vi "输入数据解析.vi"(0 "单个参数补充":dbl, 1 "从板号":dbl=1.0, 2 "主板二维码":string="BNET01", 3 "从板二维码":string="BNET01", 5 "主板引用":refnum<vi>, 7 "从板引用":refnum<vi>, 9 "主板选项":string="三级故障阀值", 11 "枚举":enum16{"主板", "从板"}(ring), 12 "快换":bool caption="快换写入") -> (4 "输出数组":dbl[][](array[numeric]), 6 "数组长度":dbl[](array[numeric]), 8 "循环次数":i32, 10 "命令":u32, 14 "名称":string[](array[string]), 15 "命令序号":u32[](array[numeric]))   [LabVIEW 2013] (continued)
                  frame "8", "钛酸锂" {
                  }
                  frame "9", "其他电池" {
                  }
                  frame "1", "磷酸铁锂", Default {
                  }
                }
                n5418 = Match Pattern(string=w14174, regular expression=w14173) -> (before substring=w14172:string, after substring=w14171:string)  [unwired: 3 out]
                n5419 = call "输入分辨率计算-EV05.vi"("1字节?"=FALSE, "数值"=w14211, "分辨率"=0.1) -> ("低字节"=w14182:dbl, "高字节1"=w14183:dbl)  [unwired: 2 in, 5 out]
                n5420 = Quotient & Remainder(x=w14190, y=w14205) -> (x-y*floor(x/y)=w14204:dbl, floor(x/y)=w14208:dbl)
                n5421 = Fract/Exp String To Number(string=w14175) -> (number=w14166:dbl)  [unwired: 4 out]
                n5422 = Quotient & Remainder(x=w14189, y=w14200) -> (x-y*floor(x/y)=w14196:dbl, floor(x/y)=w14197:dbl)
                n5423 = Quotient & Remainder(x=w14208, y=w14205) -> (x-y*floor(x/y)=w14203:dbl, floor(x/y)=w14207:dbl)
                n5424 = Fract/Exp String To Number(string=w14172) -> (number=w14165:dbl)  [unwired: 4 out]
                n5425 = Quotient & Remainder(x=w14197, y=w14200) -> (x-y*floor(x/y)=w14195:dbl, floor(x/y)=w14198:dbl)
                n5426 = call <vilib>:"Trim Whitespace.vi"("string"=w14171) -> ("trimmed string"=w14170:string)  [unwired: 1 in]
                n5427 = Quotient & Remainder(x=w14207, y=w14205) -> (x-y*floor(x/y)=w14202:dbl, floor(x/y)=w14206:dbl)
                n5428 = Quotient & Remainder(x=w14198, y=w14200) -> (x-y*floor(x/y)=w14194:dbl, floor(x/y)=w14199:dbl)
                n5429 = Quotient & Remainder(x=w14229, y=256.0) -> (x-y*floor(x/y)=w14231:dbl, floor(x/y)=w14232:dbl)
                n5430 = Fract/Exp String To Number(string=w14170) -> (number=w14164:dbl)  [unwired: 4 out]
                n5431 = Quotient & Remainder(x=w14206, y=w14205) -> (x-y*floor(x/y)=w14201:dbl)  [unwired: 1 out]
                n5432 = Quotient & Remainder(x=w14199, y=w14200) -> (x-y*floor(x/y)=w14193:dbl)  [unwired: 1 out]
                n5433 = Build Array(w14184, w14185, w14201, w14202, w14203, w14204, w14193, w14194, w14195, w14196, w14183, w14182, w14181, w14181, w14181, w14169, w14168, w14167, w14166, w14165, w14164) -> (w14180:dbl[])
                n5434 = Build Array(w14232, w14231, w14228, w14226, w14224) -> (w14230:dbl[])
                n5435 = Insert Into Array(array=w14230, new element=w14180) -> (w14213:dbl[])  [unwired: 1 in]
              }
              frame 1 {
                w14258 = 256.0 ("y")
                n5436 = Unbundle By Name(w14248) -> ("电池包组号"=w14259:string)
                n5437 = Decimal String To Number(string=w14259, default (0L)=0.0) -> (number=w14254:dbl)  [unwired: 1 in, 1 out]
                n5438 = Quotient & Remainder(x=w14254, y=w14258) -> (x-y*floor(x/y)=w14249:dbl, floor(x/y)=w14255:dbl)
                n5439 = Quotient & Remainder(x=w14255, y=w14258) -> (x-y*floor(x/y)=w14250:dbl, floor(x/y)=w14256:dbl)
                n5440 = Quotient & Remainder(x=w14256, y=w14258) -> (x-y*floor(x/y)=w14251:dbl, floor(x/y)=w14257:dbl)
                n5441 = Quotient & Remainder(x=w14257, y=w14258) -> (x-y*floor(x/y)=w14252:dbl)  [unwired: 1 out]
                n5442 = Build Array(w14252, w14251, w14250, w14249) -> (w14247:dbl[])
              }
              frame 2 {
                w14278 = 256.0 ("y")
                w14283 = 256.0 ("y")
                n5443 = Unbundle By Name(w14270) -> ("累计充电总安时"=w14267:dbl, "累计放电总安时"=w14266:dbl)
                n5444 = call "输入分辨率计算-EV05.vi"("1字节?"=TRUE, "数值 2"=w14266, "数值"=w14267, "分辨率"=0.001) -> ("高字节 2"=w14264:dbl, "高字节1"=w14265:dbl)  [unwired: 1 in, 5 out]
                n5445 = Quotient & Remainder(x=w14265, y=w14283) -> (x-y*floor(x/y)=w14282:dbl, floor(x/y)=w14286:dbl)
                n5446 = Quotient & Remainder(x=w14264, y=w14278) -> (x-y*floor(x/y)=w14274:dbl, floor(x/y)=w14275:dbl)
                n5447 = Quotient & Remainder(x=w14286, y=w14283) -> (x-y*floor(x/y)=w14281:dbl, floor(x/y)=w14285:dbl)
                n5448 = Quotient & Remainder(x=w14275, y=w14278) -> (x-y*floor(x/y)=w14273:dbl, floor(x/y)=w14276:dbl)
                n5449 = Quotient & Remainder(x=w14285, y=w14283) -> (x-y*floor(x/y)=w14280:dbl, floor(x/y)=w14284:dbl)
                n5450 = Quotient & Remainder(x=w14276, y=w14278) -> (x-y*floor(x/y)=w14272:dbl, floor(x/y)=w14277:dbl)
                n5451 = Quotient & Remainder(x=w14284, y=w14283) -> (x-y*floor(x/y)=w14279:dbl)  [unwired: 1 out]
                n5452 = Quotient & Remainder(x=w14277, y=w14278) -> (x-y*floor(x/y)=w14271:dbl)  [unwired: 1 out]
                n5453 = Build Array(w14279, w14280, w14281, w14282, w14271, w14272, w14273, w14274) -> (w14287:dbl[])
              }
              frame 3 {
                w14299 = 256.0 ("y")
                n5454 = Unbundle By Name(w14294) -> ("电池放空次数"=w14293:dbl, "电池充满次数"=w14292:dbl, "电池充电次数"=w14291:dbl)
                n5455 = Quotient & Remainder(x=w14293, y=w14299) -> (x-y*floor(x/y)=w14301:dbl, floor(x/y)=w14302:dbl)
                n5456 = Quotient & Remainder(x=w14292, y=w14299) -> (x-y*floor(x/y)=w14297:dbl, floor(x/y)=w14298:dbl)
                n5457 = Quotient & Remainder(x=w14291, y=w14299) -> (x-y*floor(x/y)=w14295:dbl, floor(x/y)=w14296:dbl)
                n5458 = Build Array(w14302, w14301, w14298, w14297, w14296, w14295) -> (w14300:dbl[])
              }
            }
          }
        }
        frame "电池包组号" {
          n5459 = Unbundle By Name(w14308) -> ("电池信息"=w14309:refnum<vi>)
          n5460 = property class="Clust (严格)"(reference=w14309) -> ("Value"=w14307:T7)  [unwired: 1 in, 2 out]
          n5461 = for {
            N: 1 -> [_]
            tunnel: [w14319] -> w14313 mode=indexing
            tunnel: [w14318] -> w14312 mode=indexing
            tunnel: [w14316] -> w14310 mode=indexing
            tunnel: w14307 -> [w14315]
            i -> [w14317]
            n5462 = case shown="0, 默认" w14317 {
              tunnel: [4 ("单个参数补充") 30 ("单个参数补充") 8 ("单个参数补充") 6 ("单个参数补充")] -> w14319
              tunnel: [2 ("命令序号") 1 ("命令序号") 4 ("命令序号") 5 ("命令序号")] -> w14318
              tunnel: [w14332 w14337 w14425 w14437] -> w14316
              tunnel: w14315 -> [w14331 w14346 w14408 w14431]
              frame 0, Default {
                w14329 = 256.0 ("y")
                n5463 = Unbundle By Name(w14331) -> ("电池包组号"=w14330:string)
                n5464 = Decimal String To Number(string=w14330, default (0L)=0.0) -> (number=w14325:dbl)  [unwired: 1 in, 1 out]
                n5465 = Quotient & Remainder(x=w14325, y=w14329) -> (x-y*floor(x/y)=w14320:dbl, floor(x/y)=w14326:dbl)
                n5466 = Quotient & Remainder(x=w14326, y=w14329) -> (x-y*floor(x/y)=w14321:dbl, floor(x/y)=w14327:dbl)
                n5467 = Quotient & Remainder(x=w14327, y=w14329) -> (x-y*floor(x/y)=w14322:dbl, floor(x/y)=w14328:dbl)
                n5468 = Quotient & Remainder(x=w14328, y=w14329) -> (x-y*floor(x/y)=w14323:dbl)  [unwired: 1 out]
                n5469 = Build Array(w14323, w14322, w14321, w14320) -> (w14332:dbl[])
              }
              frame 1 {
                w14359 = 2 ("偏移量(0)")
                w14356 = "-" ("正则表达式")
                n5470 = Unbundle By Name(w14346) -> ("电池包额定容量"=w14353:dbl, "电池包额定能量"=w14352:dbl, "电池包额定总电压"=w14347:dbl, "实际容量"=w14335:dbl)
                n5471 = Unbundle By Name(w14346) -> ("电池串联"=w14367:dbl, "电池并联"=w14366:dbl, "电池厂家"=w14365:string, "电池类型"=w14363:string, "电池生产日期"=w14361:string)
                n5472 = Match Pattern(string=w14361, regular expression=w14356) -> (before substring=w14360:string, after substring=w14357:string)  [unwired: 3 out]
                n5473 = Match Pattern(string=w14357, regular expression=w14356) -> (before substring=w14355:string, after substring=w14354:string)  [unwired: 3 out]
                n5474 = String Subset(string=w14360, offset (0)=w14359, length (rest)=w14359) -> (substring=w14358:string)
                n5475 = case shown="\"2\", \"盟固利\"" w14365 {
                  tunnel: [2 1] -> w14364
                  frame "2", "盟固利" {
                  }
                  frame "1", "普莱德", Default {
                  }
                }
                n5476 = case shown="\"9\", \"其他电池\"" w14363 {
                  tunnel: [2 3 4 5 6 7 8 9 1] -> w14362
                  frame "2", "锰酸锂" {
                  }
                  frame "3", "三元材料" {
                  }
                  frame "4", "铅酸" {
                  }
                  frame "5", "镍氢" {
                  }
                  frame "6", "钴酸锂" {
                  }
                  frame "7", "聚合物锂离子" {
                  }
                  frame "8", "钛酸锂" {
                  }
                  frame "9", "其他电池" {
                  }
                  frame "1", "磷酸铁锂", Default {
                  }
                }
                n5477 = call "输入分辨率计算-EV05.vi"("1字节?"=FALSE, "数值 2"=w14352, "数值"=w14353, "分辨率"=0.1) -> ("低字节 2"=w14342:dbl, "高字节 2"=w14343:dbl, "低字节"=w14344:dbl, "高字节1"=w14345:dbl)  [unwired: 1 in, 3 out]
                n5478 = call "输入分辨率计算-EV05.vi"("1字节?"=FALSE, "数值 2"=w14335, "数值"=w14347, "分辨率"=0.1) -> ("低字节 2"=w14338:dbl, "高字节 2"=w14339:dbl, "低字节"=w14340:dbl, "高字节1"=w14341:dbl)  [unwired: 1 in, 3 out]
                n5479 = Fract/Exp String To Number(string=w14358) -> (number=w14384:dbl)  [unwired: 1 in, 3 out]
                n5480 = Fract/Exp String To Number(string=w14355) -> (number=w14382:dbl)  [unwired: 4 out]
                n5481 = Fract/Exp String To Number(string=w14354) -> (number=w14380:dbl)  [unwired: 4 out]
                n5482 = Build Array(w14345, w14344, w14343, w14342, w14341, w14340, w14339, w14338) -> (w14336:dbl[])
                n5483 = Quotient & Remainder(x=w14367, y=256.0) -> (x-y*floor(x/y)=w14386:dbl, floor(x/y)=w14387:dbl)
                n5484 = call "二进制解析-8.6.vi"("索引"=7, "数值"=w14384) -> ("低位子数组"=w14375:i32[])  [unwired: 3 out]
                n5485 = call "二进制解析-8.6.vi"("索引"=4, "数值"=w14382) -> ("低位子数组"=w14378:i32[])  [unwired: 3 out]
                n5486 = call "二进制解析-8.6.vi"("索引"=5, "数值"=w14380) -> ("低位子数组"=w14372:i32[])  [unwired: 3 out]
                n5487 = Delete From Array(array=w14378, length=1 ("长度"), index=0 ("索引")) -> (deleted portion=w14374:i32[], array with subset deleted=w14373:i32[])
                n5488 = Insert Into Array(array=w14375, new element=w14374) -> (w14371:i32[])  [unwired: 1 in]
                n5489 = Insert Into Array(array=w14373, new element=w14372) -> (w14370:i32[])  [unwired: 1 in]
                n5490 = call "数值二进制转十进制-8.6.vi"("子数组"=w14371) -> ("十进制数值"=w14369:i32)  [unwired: 4 out]
                n5491 = call "数值二进制转十进制-8.6.vi"("子数组"=w14370) -> ("十进制数值"=w14368:i32)  [unwired: 4 out]
                n5492 = Build Array(w14387, w14386, w14366, w14364, w14362, w14369, w14368) -> (w14385:dbl[])
                n5493 = Insert Into Array(array=w14385, new element=w14336) -> (w14337:dbl[])  [unwired: 1 in]
              }
              frame 3 {
                w14416 = 256.0 ("y")
                w14421 = 256.0 ("y")
                n5494 = Unbundle By Name(w14408) -> ("累计充电总安时"=w14405:dbl, "累计放电总安时"=w14404:dbl)
                n5495 = call "输入分辨率计算-EV05.vi"("1字节?"=TRUE, "数值 2"=w14404, "数值"=w14405, "分辨率"=0.001) -> ("高字节 2"=w14402:dbl, "高字节1"=w14403:dbl)  [unwired: 1 in, 5 out]
                n5496 = Quotient & Remainder(x=w14403, y=w14421) -> (x-y*floor(x/y)=w14420:dbl, floor(x/y)=w14424:dbl)
                n5497 = Quotient & Remainder(x=w14402, y=w14416) -> (x-y*floor(x/y)=w14412:dbl, floor(x/y)=w14413:dbl)
                n5498 = Quotient & Remainder(x=w14424, y=w14421) -> (x-y*floor(x/y)=w14419:dbl, floor(x/y)=w14423:dbl)
                n5499 = Quotient & Remainder(x=w14413, y=w14416) -> (x-y*floor(x/y)=w14411:dbl, floor(x/y)=w14414:dbl)
                n5500 = Quotient & Remainder(x=w14423, y=w14421) -> (x-y*floor(x/y)=w14418:dbl, floor(x/y)=w14422:dbl)
                n5501 = Quotient & Remainder(x=w14414, y=w14416) -> (x-y*floor(x/y)=w14410:dbl, floor(x/y)=w14415:dbl)
                n5502 = Quotient & Remainder(x=w14422, y=w14421) -> (x-y*floor(x/y)=w14417:dbl)  [unwired: 1 out]
                n5503 = Quotient & Remainder(x=w14415, y=w14416) -> (x-y*floor(x/y)=w14409:dbl)  [unwired: 1 out]
                n5504 = Build Array(w14417, w14418, w14419, w14420, w14409, w14410, w14411, w14412) -> (w14425:dbl[])
              }
              frame 4 {
                w14436 = 256.0 ("y")
                n5505 = Unbundle By Name(w14431) -> ("电池放空次数"=w14430:dbl, "电池充满次数"=w14429:dbl, "电池充电次数"=w14428:dbl)
                n5506 = Quotient & Remainder(x=w14430, y=w14436) -> (x-y*floor(x/y)=w14438:dbl, floor(x/y)=w14439:dbl)
                n5507 = Quotient & Remainder(x=w14429, y=w14436) -> (x-y*floor(x/y)=w14434:dbl, floor(x/y)=w14435:dbl)
                n5508 = Quotient & Remainder(x=w14428, y=w14436) -> (x-y*floor(x/y)=w14432:dbl, floor(x/y)=w14433:dbl)
                n5509 = Build Array(w14439, w14438, w14435, w14434, w14433, w14432) -> (w14437:dbl[])
              }
            }
          }
        }
        frame "充放电安时" {
          n5510 = Unbundle By Name(w14445) -> ("电池信息"=w14446:refnum<vi>)
          n5511 = property class="Clust (严格)"(reference=w14446) -> ("Value"=w14444:T7)  [unwired: 1 in, 2 out]
          n5512 = for {
            N: 1 -> [_]
            tunnel: [w14456] -> w14450 mode=indexing
            tunnel: [w14455] -> w14449 mode=indexing
            tunnel: [w14453] -> w14447 mode=indexing
            tunnel: w14444 -> [w14452]
            i -> [w14454]
            n5513 = case shown="0, 默认" w14454 {
              tunnel: [8 ("单个参数补充") 30 ("单个参数补充") 4 ("单个参数补充") 6 ("单个参数补充")] -> w14456
              tunnel: [3 ("命令序号") 1 ("命令序号") 2 ("命令序号") 5 ("命令序号")] -> w14455
              tunnel: [w14480 w14485 w14562 w14574] -> w14453
              tunnel: w14452 -> [w14463 w14494 w14561 w14568]
              frame 0, Default {
                w14471 = 256.0 ("y")
                w14476 = 256.0 ("y")
                n5514 = Unbundle By Name(w14463) -> ("累计充电总安时"=w14460:dbl, "累计放电总安时"=w14459:dbl)
                n5515 = call "输入分辨率计算-EV05.vi"("1字节?"=TRUE, "数值 2"=w14459, "数值"=w14460, "分辨率"=0.001) -> ("高字节 2"=w14457:dbl, "高字节1"=w14458:dbl)  [unwired: 1 in, 5 out]
                n5516 = Quotient & Remainder(x=w14458, y=w14476) -> (x-y*floor(x/y)=w14475:dbl, floor(x/y)=w14479:dbl)
                n5517 = Quotient & Remainder(x=w14457, y=w14471) -> (x-y*floor(x/y)=w14467:dbl, floor(x/y)=w14468:dbl)
                n5518 = Quotient & Remainder(x=w14479, y=w14476) -> (x-y*floor(x/y)=w14474:dbl, floor(x/y)=w14478:dbl)
                n5519 = Quotient & Remainder(x=w14468, y=w14471) -> (x-y*floor(x/y)=w14466:dbl, floor(x/y)=w14469:dbl)
                n5520 = Quotient & Remainder(x=w14478, y=w14476) -> (x-y*floor(x/y)=w14473:dbl, floor(x/y)=w14477:dbl)
                n5521 = Quotient & Remainder(x=w14469, y=w14471) -> (x-y*floor(x/y)=w14465:dbl, floor(x/y)=w14470:dbl)
                n5522 = Quotient & Remainder(x=w14477, y=w14476) -> (x-y*floor(x/y)=w14472:dbl)  [unwired: 1 out]
                n5523 = Quotient & Remainder(x=w14470, y=w14471) -> (x-y*floor(x/y)=w14464:dbl)  [unwired: 1 out]
                n5524 = Build Array(w14472, w14473, w14474, w14475, w14464, w14465, w14466, w14467) -> (w14480:dbl[])
              }
              frame 1 {
                w14507 = 2 ("偏移量(0)")
                w14504 = "-" ("正则表达式")
                n5525 = Unbundle By Name(w14494) -> ("电池包额定容量"=w14501:dbl, "电池包额定能量"=w14500:dbl, "电池包额定总电压"=w14495:dbl, "实际容量"=w14483:dbl)
                n5526 = Unbundle By Name(w14494) -> ("电池串联"=w14515:dbl, "电池并联"=w14514:dbl, "电池厂家"=w14513:string, "电池类型"=w14511:string, "电池生产日期"=w14509:string)
                n5527 = Match Pattern(string=w14509, regular expression=w14504) -> (before substring=w14508:string, after substring=w14505:string)  [unwired: 3 out]
                n5528 = Match Pattern(string=w14505, regular expression=w14504) -> (before substring=w14503:string, after substring=w14502:string)  [unwired: 3 out]
                n5529 = String Subset(string=w14508, offset (0)=w14507, length (rest)=w14507) -> (substring=w14506:string)
                n5530 = case shown="\"2\", \"盟固利\"" w14513 {
                  tunnel: [2 1] -> w14512
                  frame "2", "盟固利" {
                  }
                  frame "1", "普莱德", Default {
                  }
                }
                n5531 = case shown="\"9\", \"其他电池\"" w14511 {
                  tunnel: [2 3 4 5 6 7 8 9 1] -> w14510
                  frame "2", "锰酸锂" {
                  }
                  frame "3", "三元材料" {
                  }
                  frame "4", "铅酸" {
                  }
                  frame "5", "镍氢" {
                  }
                  frame "6", "钴酸锂" {
                  }
                  frame "7", "聚合物锂离子" {
                  }
                  frame "8", "钛酸锂" {
                  }
                  frame "9", "其他电池" {
                  }
                  frame "1", "磷酸铁锂", Default {
                  }
                }
                n5532 = call "输入分辨率计算-EV05.vi"("1字节?"=FALSE, "数值 2"=w14500, "数值"=w14501, "分辨率"=0.1) -> ("低字节 2"=w14490:dbl, "高字节 2"=w14491:dbl, "低字节"=w14492:dbl, "高字节1"=w14493:dbl)  [unwired: 1 in, 3 out]
                n5533 = call "输入分辨率计算-EV05.vi"("1字节?"=FALSE, "数值 2"=w14483, "数值"=w14495, "分辨率"=0.1) -> ("低字节 2"=w14486:dbl, "高字节 2"=w14487:dbl, "低字节"=w14488:dbl, "高字节1"=w14489:dbl)  [unwired: 1 in, 3 out]
                n5534 = Fract/Exp String To Number(string=w14506) -> (number=w14532:dbl)  [unwired: 1 in, 3 out]
                n5535 = Fract/Exp String To Number(string=w14503) -> (number=w14530:dbl)  [unwired: 4 out]
                n5536 = Fract/Exp String To Number(string=w14502) -> (number=w14528:dbl)  [unwired: 4 out]
                n5537 = Build Array(w14493, w14492, w14491, w14490, w14489, w14488, w14487, w14486) -> (w14484:dbl[])
                n5538 = Quotient & Remainder(x=w14515, y=256.0) -> (x-y*floor(x/y)=w14534:dbl, floor(x/y)=w14535:dbl)
                n5539 = call "二进制解析-8.6.vi"("索引"=7, "数值"=w14532) -> ("低位子数组"=w14523:i32[])  [unwired: 3 out]
                n5540 = call "二进制解析-8.6.vi"("索引"=4, "数值"=w14530) -> ("低位子数组"=w14526:i32[])  [unwired: 3 out]
                n5541 = call "二进制解析-8.6.vi"("索引"=5, "数值"=w14528) -> ("低位子数组"=w14520:i32[])  [unwired: 3 out]
                n5542 = Delete From Array(array=w14526, length=1 ("长度"), index=0 ("索引")) -> (deleted portion=w14522:i32[], array with subset deleted=w14521:i32[])
                n5543 = Insert Into Array(array=w14523, new element=w14522) -> (w14519:i32[])  [unwired: 1 in]
                n5544 = Insert Into Array(array=w14521, new element=w14520) -> (w14518:i32[])  [unwired: 1 in]
                n5545 = call "数值二进制转十进制-8.6.vi"("子数组"=w14519) -> ("十进制数值"=w14517:i32)  [unwired: 4 out]
                n5546 = call "数值二进制转十进制-8.6.vi"("子数组"=w14518) -> ("十进制数值"=w14516:i32)  [unwired: 4 out]
                n5547 = Build Array(w14535, w14534, w14514, w14512, w14510, w14517, w14516) -> (w14533:dbl[])
                n5548 = Insert Into Array(array=w14533, new element=w14484) -> (w14485:dbl[])  [unwired: 1 in]
              }
              frame 3 {
                w14555 = 256.0 ("y")
                n5549 = Unbundle By Name(w14561) -> ("电池包组号"=w14560:string)
                n5550 = Match Pattern(string=w14560, regular expression="-" ("正则表达式")) -> (before substring=w14558:string, after substring=w14557:string)  [unwired: 3 out]
                n5551 = Fract/Exp String To Number(string=w14558) -> (number=w14556:dbl)  [unwired: 1 in, 3 out]
                n5552 = Fract/Exp String To Number(string=w14557) -> (number=w14554:dbl)  [unwired: 4 out]
                n5553 = Quotient & Remainder(x=w14554, y=w14555) -> (x-y*floor(x/y)=w14552:dbl, floor(x/y)=w14553:dbl)
                n5554 = Quotient & Remainder(x=w14556, y=w14555) -> (x-y*floor(x/y)=w14550:dbl, floor(x/y)=w14551:dbl)
                n5555 = Build Array(w14553, w14552, w14551, w14550) -> (w14562:dbl[])
              }
              frame 4 {
                w14573 = 256.0 ("y")
                n5556 = Unbundle By Name(w14568) -> ("电池放空次数"=w14567:dbl, "电池充满次数"=w14566:dbl, "电池充电次数"=w14565:dbl)
                n5557 = Quotient & Remainder(x=w14567, y=w14573) -> (x-y*floor(x/y)=w14575:dbl, floor(x/y)=w14576:dbl)
                n5558 = Quotient & Remainder(x=w14566, y=w14573) -> (x-y*floor(x/y)=w14571:dbl, floor(x/y)=w14572:dbl)
                n5559 = Quotient & Remainder(x=w14565, y=w14573) -> (x-y*floor(x/y)=w14569:dbl, floor(x/y)=w14570:dbl)
                n5560 = Build Array(w14576, w14575, w14572, w14571, w14570, w14569) -> (w14574:dbl[])
              }
            }
          }
        }
        frame "电池充放电次数" {
          n5561 = Unbundle By Name(w14582) -> ("电池信息"=w14583:refnum<vi>)
          n5562 = property class="Clust (严格)"(reference=w14583) -> ("Value"=w14581:T7)  [unwired: 1 in, 2 out]
          n5563 = for {
            N: 1 -> [_]
            tunnel: [w14593] -> w14587 mode=indexing
            tunnel: [w14592] -> w14586 mode=indexing
            tunnel: [w14590] -> w14584 mode=indexing
            tunnel: w14581 -> [w14589]
            i -> [w14591]
            n5564 = case shown="0, 默认" w14591 {
              tunnel: [6 ("单个参数补充") 30 ("单个参数补充") 4 ("单个参数补充") 8 ("单个参数补充")] -> w14593
              tunnel: [4 ("命令序号") 1 ("命令序号") 2 ("命令序号") 3 ("命令序号")] -> w14592
              tunnel: [w14603 w14610 w14687 w14713] -> w14590
              tunnel: w14589 -> [w14597 w14619 w14686 w14696]
              frame 0, Default {
                w14602 = 256.0 ("y")
                n5565 = Unbundle By Name(w14597) -> ("电池放空次数"=w14596:dbl, "电池充满次数"=w14595:dbl, "电池充电次数"=w14594:dbl)
                n5566 = Quotient & Remainder(x=w14596, y=w14602) -> (x-y*floor(x/y)=w14604:dbl, floor(x/y)=w14605:dbl)
                n5567 = Quotient & Remainder(x=w14595, y=w14602) -> (x-y*floor(x/y)=w14600:dbl, floor(x/y)=w14601:dbl)
                n5568 = Quotient & Remainder(x=w14594, y=w14602) -> (x-y*floor(x/y)=w14598:dbl, floor(x/y)=w14599:dbl)
                n5569 = Build Array(w14605, w14604, w14601, w14600, w14599, w14598) -> (w14603:dbl[])
              }
              frame 1 {
                w14632 = 2 ("偏移量(0)")
                w14629 = "-" ("正则表达式")
                n5570 = Unbundle By Name(w14619) -> ("电池包额定容量"=w14626:dbl, "电池包额定能量"=w14625:dbl, "电池包额定总电压"=w14620:dbl, "实际容量"=w14608:dbl)
                n5571 = Unbundle By Name(w14619) -> ("电池串联"=w14640:dbl, "电池并联"=w14639:dbl, "电池厂家"=w14638:string, "电池类型"=w14636:string, "电池生产日期"=w14634:string)
                n5572 = Match Pattern(string=w14634, regular expression=w14629) -> (before substring=w14633:string, after substring=w14630:string)  [unwired: 3 out]
                n5573 = Match Pattern(string=w14630, regular expression=w14629) -> (before substring=w14628:string, after substring=w14627:string)  [unwired: 3 out]
                n5574 = String Subset(string=w14633, offset (0)=w14632, length (rest)=w14632) -> (substring=w14631:string)
                n5575 = case shown="\"2\", \"盟固利\"" w14638 {
                  tunnel: [2 1] -> w14637
                  frame "2", "盟固利" {
                  }
                  frame "1", "普莱德", Default {
                  }
                }
                n5576 = case shown="\"9\", \"其他电池\"" w14636 {
                  tunnel: [2 3 4 5 6 7 8 9 1] -> w14635
                  frame "2", "锰酸锂" {
                  }
                  frame "3", "三元材料" {
                  }
                  frame "4", "铅酸" {
                  }
                  frame "5", "镍氢" {
                  }
                  frame "6", "钴酸锂" {
                  }
                  frame "7", "聚合物锂离子" {
                  }
                  frame "8", "钛酸锂" {
                  }
                  frame "9", "其他电池" {
                  }
                  frame "1", "磷酸铁锂", Default {
                  }
                }
                n5577 = call "输入分辨率计算-EV05.vi"("1字节?"=FALSE, "数值 2"=w14625, "数值"=w14626, "分辨率"=0.1) -> ("低字节 2"=w14615:dbl, "高字节 2"=w14616:dbl, "低字节"=w14617:dbl, "高字节1"=w14618:dbl)  [unwired: 1 in, 3 out]
                n5578 = call "输入分辨率计算-EV05.vi"("1字节?"=FALSE, "数值 2"=w14608, "数值"=w14620, "分辨率"=0.1) -> ("低字节 2"=w14611:dbl, "高字节 2"=w14612:dbl, "低字节"=w14613:dbl, "高字节1"=w14614:dbl)  [unwired: 1 in, 3 out]
                n5579 = Fract/Exp String To Number(string=w14631) -> (number=w14657:dbl)  [unwired: 1 in, 3 out]
                n5580 = Fract/Exp String To Number(string=w14628) -> (number=w14655:dbl)  [unwired: 4 out]
                n5581 = Fract/Exp String To Number(string=w14627) -> (number=w14653:dbl)  [unwired: 4 out]
                n5582 = Build Array(w14618, w14617, w14616, w14615, w14614, w14613, w14612, w14611) -> (w14609:dbl[])
                n5583 = Quotient & Remainder(x=w14640, y=256.0) -> (x-y*floor(x/y)=w14659:dbl, floor(x/y)=w14660:dbl)
                n5584 = call "二进制解析-8.6.vi"("索引"=7, "数值"=w14657) -> ("低位子数组"=w14648:i32[])  [unwired: 3 out]
                n5585 = call "二进制解析-8.6.vi"("索引"=4, "数值"=w14655) -> ("低位子数组"=w14651:i32[])  [unwired: 3 out]
                n5586 = call "二进制解析-8.6.vi"("索引"=5, "数值"=w14653) -> ("低位子数组"=w14645:i32[])  [unwired: 3 out]
                n5587 = Delete From Array(array=w14651, length=1 ("长度"), index=0 ("索引")) -> (deleted portion=w14647:i32[], array with subset deleted=w14646:i32[])
                n5588 = Insert Into Array(array=w14648, new element=w14647) -> (w14644:i32[])  [unwired: 1 in]
                n5589 = Insert Into Array(array=w14646, new element=w14645) -> (w14643:i32[])  [unwired: 1 in]
                n5590 = call "数值二进制转十进制-8.6.vi"("子数组"=w14644) -> ("十进制数值"=w14642:i32)  [unwired: 4 out]
                n5591 = call "数值二进制转十进制-8.6.vi"("子数组"=w14643) -> ("十进制数值"=w14641:i32)  [unwired: 4 out]
                n5592 = Build Array(w14660, w14659, w14639, w14637, w14635, w14642, w14641) -> (w14658:dbl[])
                n5593 = Insert Into Array(array=w14658, new element=w14609) -> (w14610:dbl[])  [unwired: 1 in]
              }
              frame 3 {
                w14680 = 256.0 ("y")
                n5594 = Unbundle By Name(w14686) -> ("电池包组号"=w14685:string)
                n5595 = Match Pattern(string=w14685, regular expression="-" ("正则表达式")) -> (before substring=w14683:string, after substring=w14682:string)  [unwired: 3 out]
                n5596 = Fract/Exp String To Number(string=w14683) -> (number=w14681:dbl)  [unwired: 1 in, 3 out]
                n5597 = Fract/Exp String To Number(string=w14682) -> (number=w14679:dbl)  [unwired: 4 out]
                n5598 = Quotient & Remainder(x=w14679, y=w14680) -> (x-y*floor(x/y)=w14677:dbl, floor(x/y)=w14678:dbl)
                n5599 = Quotient & Remainder(x=w14681, y=w14680) -> (x-y*floor(x/y)=w14675:dbl, floor(x/y)=w14676:dbl)
                n5600 = Build Array(w14678, w14677, w14676, w14675) -> (w14687:dbl[])
              }
              frame 4 {
                w14704 = 256.0 ("y")
                w14709 = 256.0 ("y")
                n5601 = Unbundle By Name(w14696) -> ("累计充电总安时"=w14693:dbl, "累计放电总安时"=w14692:dbl)
                n5602 = call "输入分辨率计算-EV05.vi"("1字节?"=TRUE, "数值 2"=w14692, "数值"=w14693, "分辨率"=0.001) -> ("高字节 2"=w14690:dbl, "高字节1"=w14691:dbl)  [unwired: 1 in, 5 out]
                n5603 = Quotient & Remainder(x=w14691, y=w14709) -> (x-y*floor(x/y)=w14708:dbl, floor(x/y)=w14712:dbl)
                n5604 = Quotient & Remainder(x=w14690, y=w14704) -> (x-y*floor(x/y)=w14700:dbl, floor(x/y)=w14701:dbl)
                n5605 = Quotient & Remainder(x=w14712, y=w14709) -> (x-y*floor(x/y)=w14707:dbl, floor(x/y)=w14711:dbl)
                n5606 = Quotient & Remainder(x=w14701, y=w14704) -> (x-y*floor(x/y)=w14699:dbl, floor(x/y)=w14702:dbl)
                n5607 = Quotient & Remainder(x=w14711, y=w14709) -> (x-y*floor(x/y)=w14706:dbl, floor(x/y)=w14710:dbl)
                n5608 = Quotient & Remainder(x=w14702, y=w14704) -> (x-y*floor(x/y)=w14698:dbl, floor(x/y)=w14703:dbl)
                n5609 = Quotient & Remainder(x=w14710, y=w14709) -> (x-y*floor(x/y)=w14705:dbl)  [unwired: 1 out]
                n5610 = Quotient & Remainder(x=w14703, y=w14704) -> (x-y*floor(x/y)=w14697:dbl)  [unwired: 1 out]
                n5611 = Build Array(w14705, w14706, w14707, w14708, w14697, w14698, w14699, w14700) -> (w14713:dbl[])
              }
            }
          }
        }
        frame "历史信息" {
          n5612 = disable-structure shown="禁用" {
            disable-tunnel: [u32 163 ("命令序号") _] -> w14720
            disable-tunnel: [w14725 _] -> w14719
            disable-tunnel: [w14724 _] -> w14718
            disable-tunnel: w14717 -> [w14723 _]
            disable-tunnel: [w14721 _] -> w14716
            frame Disabled {
              n5613 = for {
                N: 4 -> [_]
                tunnel: [w14731] -> w14725 mode=indexing
                tunnel: [w14730] -> w14724 mode=indexing
                tunnel: w14723 -> [w14728]
                tunnel: [w14727] -> w14721 mode=indexing
                i -> [w14729]
                n5614 = case shown="0, 默认" w14729 {
                  tunnel: [14 ("单个参数补充") 9 ("单个参数补充") 12 ("单个参数补充") 12 ("单个参数补充")] -> w14731
                  tunnel: [1 ("命令序号") 2 ("命令序号") 3 ("命令序号") 4 ("命令序号")] -> w14730
                  tunnel: w14728 -> [w14739 w14774 w14805 w14833]
                  tunnel: [w14733 w14768 w14799 w14831] -> w14727
                  frame 0, Default {
                    n5615 = Index Array(array=w14739, index (col)=22 ("禁用的索引 (列)")) -> (element=w14738)  [unwired: 1 in]
                    n5616 = Array Subset(array=w14738, index=0 ("索引"), length=7 ("长度")) -> (w14735:void[])
                    n5617 = Fract/Exp String To Number(string=w14735) -> (number=w14734:dbl[])  [unwired: 1 in, 3 out]
                    n5618 = for {
                      tunnel: w14734 -> [w14751] mode=indexing
                      shift-right: [w14746] -> w14733
                      shift-left: dbl[] [] -> [w14745]
                      i -> [w14752]
                      n5619 = case shown="6" w14752 {
                        tunnel: [0.001 ("分辨率") 0.001 ("分辨率") 1.0 ("分辨率") 0.001 ("分辨率") 0.001 ("分辨率") 0.1 ("分辨率") 0.1 ("分辨率")] -> w14744
                        tunnel: [0.0 ("分辨率") 0.0 ("分辨率") 0.0 ("分辨率") 0.0 ("分辨率") 0.0 ("分辨率") 0.0 ("分辨率") 0.0 ("分辨率")] -> w14743
                        frame 0, Default {
                        }
                        frame 1 {
                        }
                        frame 2 {
                        }
                        frame 3 {
                        }
                        frame 4 {
                        }
                        frame 5 {
                        }
                        frame 6 {
                        }
                      }
                      n5620 = call "输入分辨率计算-EV05.vi"("1字节?"=FALSE, "数值"=w14751, "偏移量"=w14743, "分辨率"=w14744) -> ("低字节"=w14748:dbl, "高字节1"=w14749:dbl)  [unwired: 1 in, 5 out]
                      n5621 = Build Array(w14749, w14748) -> (w14747:dbl[])
                      n5622 = Insert Into Array(array=w14745, new element=w14747) -> (w14746:dbl[])  [unwired: 1 in]
                    }
                  }
                  frame 1 {
                    n5623 = Index Array(array=w14774, index (col)=22 ("禁用的索引 (列)")) -> (element=w14773)  [unwired: 1 in]
                    n5624 = Array Subset(array=w14773, index=8 ("索引"), length=9 ("长度")) -> (w14770:void[])
                    n5625 = Fract/Exp String To Number(string=w14770) -> (number=w14769:dbl[])  [unwired: 1 in, 3 out]
                    n5626 = for {
                      tunnel: w14769 -> [w14784] mode=indexing
                      shift-right: [w14782] -> w14768
                      shift-left: dbl[] [] -> [w14781]
                      i -> [w14785]
                      n5627 = case shown="0, 默认" w14785 {
                        tunnel: [1.0 ("分辨率") 1.0 ("分辨率") 1.0 ("分辨率") 1.0 ("分辨率") 1.0 ("分辨率") 1.0 ("分辨率")] -> w14780
                        tunnel: [-40.0 ("分辨率") -40.0 ("分辨率") 0.0 ("分辨率") -40.0 ("分辨率") -40.0 ("分辨率") 0.0 ("分辨率")] -> w14779
                        frame 0, Default {
                        }
                        frame 1 {
                        }
                        frame 2 {
                        }
                        frame 3 {
                        }
                        frame 4 {
                        }
                        frame 5..8 {
                        }
                      }
                      n5628 = call "输入分辨率计算-EV05.vi"("1字节?"=TRUE, "数值"=w14784, "偏移量"=w14779, "分辨率"=w14780) -> ("高字节1"=w14778:dbl)  [unwired: 1 in, 6 out]
                      n5629 = Insert Into Array(array=w14781, new element=w14778) -> (w14782:dbl[])  [unwired: 1 in]
                    }
                  }
                  frame 2 {
                    n5630 = Index Array(array=w14805, index (col)=22 ("禁用的索引 (列)")) -> (element=w14804)  [unwired: 1 in]
                    n5631 = Array Subset(array=w14804, index=17 ("索引"), length=6 ("长度")) -> (w14801:void[])
                    n5632 = Fract/Exp String To Number(string=w14801) -> (number=w14800:dbl[])  [unwired: 1 in, 3 out]
                    n5633 = for {
                      tunnel: w14800 -> [w14817] mode=indexing
                      shift-right: [w14812] -> w14799
                      shift-left: dbl[] [] -> [w14811]
                      i -> [w14818]
                      n5634 = case shown="4, 5" w14818 {
                        tunnel: [0.01 ("分辨率") 0.01 ("分辨率") 0.1 ("分辨率") 0.1 ("分辨率") 1.0 ("分辨率")] -> w14810
                        tunnel: [-300.0 ("分辨率") -300.0 ("分辨率") -3000.0 ("分辨率") -3000.0 ("分辨率") 0.0 ("分辨率")] -> w14809
                        frame 0, Default {
                        }
                        frame 1 {
                        }
                        frame 2 {
                        }
                        frame 3 {
                        }
                        frame 4, 5 {
                        }
                      }
                      n5635 = call "输入分辨率计算-EV05.vi"("1字节?"=FALSE, "数值"=w14817, "偏移量"=w14809, "分辨率"=w14810) -> ("低字节"=w14814:dbl, "高字节1"=w14815:dbl)  [unwired: 1 in, 5 out]
                      n5636 = Build Array(w14815, w14814) -> (w14813:dbl[])
                      n5637 = Insert Into Array(array=w14811, new element=w14813) -> (w14812:dbl[])  [unwired: 1 in]
                    }
                  }
                  frame 3 {
                    w14839 = 256.0 ("y")
                    w14851 = 256.0 ("y")
                    w14856 = 256.0 ("y")
                    n5638 = Index Array(array=w14833, index (col)=22 ("禁用的索引 (列)")) -> (element=w14866)  [unwired: 1 in]
                    n5639 = Index Array(array=w14866, index #1=23 ("索引"), index #2=24 ("索引"), index #3=25 ("索引")) -> (element #1=w14832, element #2=w14861, element #3=w14860)
                    n5640 = Fract/Exp String To Number(string=w14861) -> (number=w14847:dbl)  [unwired: 1 in, 3 out]
                    n5641 = Fract/Exp String To Number(string=w14832) -> (number=w14862:dbl)  [unwired: 1 in, 3 out]
                    n5642 = Fract/Exp String To Number(string=w14860) -> (number=w14838:dbl)  [unwired: 4 out]
                    n5643 = Quotient & Remainder(x=w14862, y=w14856) -> (x-y*floor(x/y)=w14855:dbl, floor(x/y)=w14859:dbl)
                    n5644 = Quotient & Remainder(x=w14847, y=w14851) -> (x-y*floor(x/y)=w14846:dbl, floor(x/y)=w14848:dbl)
                    n5645 = Quotient & Remainder(x=w14838, y=w14839) -> (x-y*floor(x/y)=w14837:dbl, floor(x/y)=w14842:dbl)
                    n5646 = Quotient & Remainder(x=w14859, y=w14856) -> (x-y*floor(x/y)=w14854:dbl, floor(x/y)=w14858:dbl)
                    n5647 = Quotient & Remainder(x=w14848, y=w14851) -> (x-y*floor(x/y)=w14845:dbl, floor(x/y)=w14849:dbl)
                    n5648 = Quotient & Remainder(x=w14842, y=w14839) -> (x-y*floor(x/y)=w14836:dbl, floor(x/y)=w14841:dbl)
                    n5649 = Quotient & Remainder(x=w14858, y=w14856) -> (x-y*floor(x/y)=w14853:dbl, floor(x/y)=w14857:dbl)
                    n5650 = Quotient & Remainder(x=w14849, y=w14851) -> (x-y*floor(x/y)=w14844:dbl, floor(x/y)=w14850:dbl)
                    n5651 = Quotient & Remainder(x=w14841, y=w14839) -> (x-y*floor(x/y)=w14835:dbl, floor(x/y)=w14840:dbl)
                    n5652 = Quotient & Remainder(x=w14857, y=w14856) -> (x-y*floor(x/y)=w14852:dbl)  [unwired: 1 out]
                    n5653 = Quotient & Remainder(x=w14850, y=w14851) -> (x-y*floor(x/y)=w14843:dbl)  [unwired: 1 out]
                    n5654 = Quotient & Remainder(x=w14840, y=w14839) -> (x-y*floor(x/y)=w14834:dbl)  [unwired: 1 out]
                    n5655 = Build Array(w14852, w14853, w14854, w14855, w14843, w14844, w14845, w14846, w14834, w14835, w14836, w14837) -> (w14831:dbl[])
                  }
                }
              }
            }
            frame Enabled {
            }
          }
        }
      }
    }
    frame "从板" {
      n5656 = property class="Clust (严格)"(reference="从板引用") -> ("Value"=w14870:T1)  [unwired: 1 in, 2 out]
      n5657 = case shown="\"电压个数\"" w14879 {
        tunnel: w14870 -> [_ w14889 w14899 w14936 w15072 w15100 w15138 w15174 w15354 w15529 w15704 w15879 w16054 w16229 w16404 w16582 w16648 w16750 w16852 w16954 w17056 w17158 w17260 w17362 w17464 w17566 w17668 w17770 w17872 w17974 w18076 w18178 w18280 w18382 w18484 w18574 w18664 w18754 w18819 w18885 w19086 w19185 w19284 w19382 w19582 w19725 w19868 w20011 w20154 _ w20312]
        tunnel: [_ w14886 w14902 w14939 w15075 w15103 w15141 w15177 w15357 w15532 w15707 w15882 w16057 w16232 w16407 w16584 w16650 w16752 w16854 w16956 w17058 w17160 w17262 w17364 w17466 w17568 w17670 w17772 w17874 w17976 w18078 w18180 w18282 w18384 w18486 w18576 w18666 w18756 w18821 w18884 w19085 w19184 w19283 w19381 w19581 w19724 w19867 w20010 w20153 w20297 w20311] -> w14878
        tunnel: [_ u32 32 ("命令序号") u32 32 ("命令序号") u32 32 ("命令序号") u32 32 ("命令序号") u32 32 ("命令序号") u32 32 ("命令序号") u32 32 ("命令序号") u32 32 ("命令序号") u32 32 ("命令序号") u32 32 ("命令序号") u32 32 ("命令序号") u32 32 ("命令序号") u32 32 ("命令序号") u32 32 ("命令序号") u32 34 ("命令序号") u32 34 ("命令序号") u32 34 ("命令序号") u32 34 ("命令序号") u32 34 ("命令序号") u32 34 ("命令序号") u32 34 ("命令序号") u32 34 ("命令序号") u32 34 ("命令序号") u32 34 ("命令序号") u32 34 ("命令序号") u32 34 ("命令序号") u32 34 ("命令序号") u32 34 ("命令序号") u32 34 ("命令序号") u32 34 ("命令序号") u32 34 ("命令序号") u32 34 ("命令序号") u32 34 ("命令序号") u32 34 ("命令序号") u32 34 ("命令序号") u32 34 ("命令序号") u32 34 ("命令序号") u32 34 ("命令序号") w18882 u32 38 ("命令序号") u32 38 ("命令序号") u32 38 ("命令序号") w19379 w19579 w19722 w19865 w20008 w20151 u32 42 ("命令序号") w20309] -> w14877
        tunnel: [_ u32[] [6] w14900 w14937 w15073 w15101 w15139 w15175 w15355 w15530 w15705 w15880 w16055 w16230 w16405 u32[] [1] u32[] [1] u32[] [2] u32[] [3] u32[] [1] u32[] [2] u32[] [3] u32[] [1] u32[] [2] u32[] [3] u32[] [1] u32[] [2] u32[] [3] u32[] [1] u32[] [2] u32[] [3] u32[] [1] u32[] [2] u32[] [3] u32[] [1] u32[] [2] u32[] [3] u32[] [2] u32[] [3] w18886 w19087 w19186 w19285 w19383 w19583 w19726 w19869 w20012 w20155 w20294 w20313] -> w14876
        tunnel: [_ dbl[] [1.0] w14901 w14938 w15074 w15102 w15140 w15176 w15356 w15531 w15706 w15881 w16056 w16231 w16406 dbl[] [15.0] dbl[] [15.0] dbl[] [15.0] dbl[] [15.0] dbl[] [15.0] dbl[] [15.0] dbl[] [15.0] dbl[] [15.0] dbl[] [15.0] dbl[] [15.0] dbl[] [15.0] dbl[] [15.0] dbl[] [15.0] dbl[] [15.0] dbl[] [15.0] dbl[] [15.0] dbl[] [15.0] dbl[] [15.0] dbl[] [15.0] dbl[] [15.0] dbl[] [15.0] dbl[] [15.0] dbl[] [15.0] dbl[] [15.0] w18887 w19088 w19187 w19286 w19384 w19584 w19727 w19870 w20013 w20156 w20295 w20314] -> w14875
        tunnel: w14874 -> [_ _ _ _ _ _ _ w15178 w15358 w15533 w15708 w15883 w16058 w16233 w16408 _ _ _ _ _ _ _ _ _ _ _ _ _ _ _ _ _ _ _ _ _ _ _ _ _ _ _ _ _ _ _ _ _ _ _ _]
        tunnel: w14873 -> [_ _ _ _ _ _ _ _ _ _ _ _ _ _ _ _ _ _ _ _ _ _ _ _ _ _ _ _ _ _ _ _ _ _ _ _ _ _ _ w18883 _ _ _ w19380 w19580 w19723 w19866 w20009 w20152 _ w20310]
        tunnel: w14872 -> [_ w14882 _ w14934 _ _ _ _ _ _ _ _ _ _ _ _ _ _ _ _ _ _ _ _ _ _ _ _ _ _ _ _ _ _ _ _ _ _ _ _ _ _ _ _ _ _ _ _ _ _ _]
        tunnel: [_ 1 1 5 1 1 1 1 1 1 1 1 1 1 1 1 1 1 1 1 1 1 1 1 1 1 1 1 1 1 1 1 1 1 1 1 1 1 1 w18881 w19083 w19182 w19281 w19378 1 1 1 1 1 1 1] -> w14869
        tunnel: [_ string[] ["从板号"] string[] ["电压起始值"] w14933 string[] ["通道电压节数"] string[] ["保险位置"] string[] ["温度起始值"] string[] ["加热控制参数"] string[] ["加热控制参数"] string[] ["加热控制参数"] string[] ["加热控制参数"] string[] ["加热控制参数"] string[] ["加热控制参数"] string[] ["加热控制参数"] string[] ["加热控制参数"] string[] ["一级故障阀值"] string[] ["一级故障阀值"] string[] ["二级故障阀值"] string[] ["三级故障阀值"] string[] ["一级故障阀值"] string[] ["二级故障阀值"] string[] ["三级故障阀值"] string[] ["一级故障阀值"] string[] ["二级故障阀值"] string[] ["三级故障阀值"] string[] ["一级故障阀值"] string[] ["二级故障阀值"] string[] ["三级故障阀值"] string[] ["一级故障阀值"] string[] ["二级故障阀值"] string[] ["三级故障阀值"] string[] ["一级故障阀值"] string[] ["二级故障阀值"] string[] ["三级故障阀值"] string[] ["一级故障阀值"] string[] ["二级故障阀值"] string[] ["三级故障阀值"] string[] ["二级故障阀值"] string[] ["三级故障阀值"] w18880 w19082 w19181 w19280 w19377 string[] ["电池包序号"] string[] ["充放电安时"] string[] ["充电次数时间"] string[] ["SOC"] string[] ["车牌号"] w20296 string[] ["充电参数"]] -> w14868
        frame "假", Default {
        }
        frame "从板号" {
          n5658 = disable-structure shown="启用" {
            disable-tunnel: w14889 -> [w14895 _]
            disable-tunnel: [w14890 w14896] -> w14888
            disable-tunnel: w14882 -> [_ w14896]
            frame Disabled {
              n5659 = Index Array(array=w14895, index (col)=4 ("禁用的索引 (列)")) -> (element=w14893)  [unwired: 1 in]
              n5660 = Index Array(array=w14893, index=1 ("索引")) -> (element=w14891)
              n5661 = Fract/Exp String To Number(string=w14891) -> (number=w14890:dbl)  [unwired: 4 out]
            }
            frame Enabled {
            }
          }
          n5662 = Build Array(w14888) -> (w14887:dbl[])
          n5663 = Build Array(w14887) -> (w14886:dbl[][])
        }
        frame "电压个数" {
          n5664 = for {
            N: 1 -> [_]
            tunnel: [w14908] -> w14902 mode=indexing
            tunnel: [w14907] -> w14901 mode=indexing
            tunnel: [w14906] -> w14900 mode=indexing
            tunnel: w14899 -> [w14905]
            i -> [w14909]
            n5665 = case shown="0, 默认" w14909 {
              tunnel: w14905 -> [w14917]
              tunnel: [w14912] -> w14908
              tunnel: [4.0 ("y")] -> w14907
              tunnel: [u32 1 ("命令序号")] -> w14906
              frame 0, Default {
                n5666 = Unbundle By Name(w14917) -> ("项目信息 2"=w14918:refnum<vi>)
                n5667 = property class="Tbl (严格)"(reference=w14918) -> ("Value"=w14916:string[][])  [unwired: 1 in, 2 out]
                n5668 = Index Array(array=w14916, index (col)=1 ("禁用的索引 (列)")) -> (element=w14920:string[])  [unwired: 1 in]
                n5669 = Array Subset(array=w14920, index=0 ("索引"), length=2.0 ("y")) -> (w14921:string[])
                n5670 = Fract/Exp String To Number(string=w14921) -> (number=w14914:dbl[])  [unwired: 4 out]
                n5671 = for {
                  N: 1 -> [_]
                  tunnel: w14914 -> [w14932] mode=indexing
                  shift-right: [w14927] -> w14912
                  shift-left: dbl[] [] -> [w14926]
                  n5672 = Quotient & Remainder(x=w14932, y=256.0) -> (x-y*floor(x/y)=w14929:dbl, floor(x/y)=w14930:dbl)
                  n5673 = Build Array(w14930, w14929, 0.0 ("元素"), 1.0 ("元素")) -> (w14928:dbl[])
                  n5674 = Insert Into Array(array=w14926, new element=w14928) -> (w14927:dbl[])  [unwired: 1 in]
                }
              }
            }
          }
        }
        frame "从板信息" {
          n5675 = for {
            N: 5 -> [_]
            tunnel: [w14947] -> w14939 mode=indexing
            tunnel: [w14946] -> w14938 mode=indexing
            tunnel: [w14945] -> w14937 mode=indexing
            tunnel: w14936 -> [w14944]
            tunnel: w14934 -> [w14943]
            tunnel: [w14942] -> w14933 mode=indexing
            i -> [w14948]
            n5676 = case shown="4" w14948 {
              tunnel: w14944 -> [w14957 w14979 w14997 w15023 w15050 _]
              tunnel: [w14952 w14974 w14991 w15021 w15049 w15066] -> w14947
              tunnel: [4.0 ("y") 20.0 ("y") 10.0 ("y") 4.0 ("y") 7.0 ("y") 1.0 ("y")] -> w14946
              tunnel: [u32 1 ("命令序号") u32 2 ("命令序号") u32 3 ("命令序号") u32 4 ("命令序号") u32 5 ("命令序号") u32 6 ("命令序号")] -> w14945
              tunnel: w14943 -> [_ _ _ _ _ w15069]
              tunnel: ["电压起始值" "通道电压节数" "保险位置" "温度起始值" "加热控制参数" "从板号"] -> w14942
              frame 0, Default {
                # "起始位置改为1"
                n5677 = Unbundle By Name(w14957) -> ("项目信息 2"=w14958:refnum<vi>)
                n5678 = property class="Tbl (严格)"(reference=w14958) -> ("Value"=w14956:string[][])  [unwired: 1 in, 2 out]
                n5679 = Index Array(array=w14956, index (col)=1 ("禁用的索引 (列)")) -> (element=w14960:string[])  [unwired: 1 in]
                n5680 = Array Subset(array=w14960, index=0 ("索引"), length=1.0 ("y")) -> (w14961:string[])
                n5681 = Fract/Exp String To Number(string=w14961) -> (number=w14954:dbl[])  [unwired: 4 out]
                n5682 = for {
                  N: 1 -> [_]
                  tunnel: w14954 -> [w14972] mode=indexing
                  shift-right: [w14967] -> w14952
                  shift-left: dbl[] [] -> [w14966]
                  n5683 = Quotient & Remainder(x=w14972, y=256.0) -> (x-y*floor(x/y)=w14969:dbl, floor(x/y)=w14970:dbl)
                  n5684 = Build Array(w14970, w14969, 0.0 ("元素"), 1.0 ("元素")) -> (w14968:dbl[])
                  n5685 = Insert Into Array(array=w14966, new element=w14968) -> (w14967:dbl[])  [unwired: 1 in]
                }
              }
              frame 1 {
                n5686 = Unbundle By Name(w14979) -> ("项目信息 2"=w14982:refnum<vi>)
                n5687 = property class="Tbl (严格)"(reference=w14982) -> ("Value"=w14981:string[][])  [unwired: 1 in, 2 out]
                n5688 = Index Array(array=w14981, index (col)=1 ("禁用的索引 (列)")) -> (element=w14983:string[])  [unwired: 1 in]
                n5689 = Array Subset(array=w14983, index=22 ("索引"), length=5.0 ("y")) -> (w14984:string[])
                n5690 = Fract/Exp String To Number(string=w14984) -> (number=w14975:dbl[])  [unwired: 4 out]
                n5691 = for {
                  N: 20 -> [_]
                  tunnel: w14975 -> [w14988] mode=indexing
                  tunnel: [w14987] -> w14974 mode=indexing
                  w14989 = 12.0 ("y")
                  n5692 = Greater?(x=w14988, y=w14989) -> (0:w14990:bool)
                  n5693 = Select(t=w14989, s=w14990, f=w14988) -> (s? t:f=w14987:dbl)
                }
              }
              frame 2 {
                n5694 = Unbundle By Name(w14997) -> ("项目信息 2"=w15000:refnum<vi>)
                n5695 = property class="Tbl (严格)"(reference=w15000) -> ("Value"=w14999:string[][])  [unwired: 1 in, 2 out]
                n5696 = Index Array(array=w14999, index (col)=1 ("禁用的索引 (列)")) -> (element=w15001:string[])  [unwired: 1 in]
                n5697 = Array Subset(array=w15001, index=2 ("索引"), length=20.0 ("y")) -> (w15002:string[])
                n5698 = Fract/Exp String To Number(string=w15002) -> (number=w14993:dbl[])  [unwired: 4 out]
                n5699 = for {
                  N: 10 -> [_]
                  tunnel: w14993 -> [w15014]
                  tunnel: [w15005] -> w14991 mode=indexing
                  i -> [w15016]
                  w15009 = 4 ("索引")
                  n5700 = Multiply(x=w15016, y=2) -> (x*y=w15013:i32)
                  n5701 = Increment(x=w15013) -> (x+1=w15012:i32)
                  n5702 = Index Array(array=w15014, index #1=w15013, index #2=w15012) -> (element #1=w15011:dbl, element #2=w15010:dbl)
                  n5703 = call "二进制解析-8.6.vi"("索引"=w15009, "数值"=w15011) -> ("低位子数组"=w15008:i32[])  [unwired: 1 in, 2 out]
                  n5704 = call "二进制解析-8.6.vi"("索引"=w15009, "数值"=w15010) -> ("低位子数组"=w15007:i32[])  [unwired: 1 in, 2 out]
                  n5705 = Insert Into Array(array=w15008, new element=w15007) -> (w15006:i32[])  [unwired: 1 in]
                  n5706 = call "数值二进制转十进制-8.6.vi"("子数组"=w15006) -> ("十进制数值"=w15005:i32)  [unwired: 4 in]
                }
              }
              frame 3 {
                n5707 = Unbundle By Name(w15023) -> ("项目信息 2"=w15027:refnum<vi>)
                n5708 = property class="Tbl (严格)"(reference=w15027) -> ("Value"=w15026:string[][])  [unwired: 1 in, 2 out]
                n5709 = Index Array(array=w15026, index (col)=1 ("禁用的索引 (列)")) -> (element=w15028:string[])  [unwired: 1 in]
                n5710 = Array Subset(array=w15028, index=1 ("索引"), length=1.0 ("y")) -> (w15029:string[])
                n5711 = Fract/Exp String To Number(string=w15029) -> (number=w15025:dbl[])  [unwired: 4 out]
                n5712 = for {
                  N: 1 -> [_]
                  tunnel: w15025 -> [w15040] mode=indexing
                  shift-right: [w15035] -> w15021
                  shift-left: dbl[] [] -> [w15034]
                  n5713 = Quotient & Remainder(x=w15040, y=256.0) -> (x-y*floor(x/y)=w15037:dbl, floor(x/y)=w15038:dbl)
                  n5714 = Build Array(w15038, w15037, 0.0 ("元素"), 1.0 ("元素")) -> (w15036:dbl[])
                  n5715 = Insert Into Array(array=w15034, new element=w15036) -> (w15035:dbl[])  [unwired: 1 in]
                }
              }
              frame 4 {
                n5716 = Unbundle By Name(w15050) -> ("加热控制参数"=w15064:refnum<vi>)
                n5717 = property class="Clust (严格)"(reference=w15064) -> ("Value"=w15063:T5)  [unwired: 1 in, 2 out]
                n5718 = Unbundle(w15063) -> ("风机开启温度"=w15058:dbl, "风机关闭温度"=w15057:dbl, "加热开启温度"=w15054:dbl, "加热关闭温度"=w15053:dbl, "风机开启温差"=w15045:dbl, "风机关闭温差"=w15043:dbl, "加热关闭温差"=w15041:dbl)
                n5719 = call "输入分辨率计算-EV05.vi"("1字节?"=TRUE, "数值 2"=w15053, "数值"=w15054, "偏移量"=-40.0, "分辨率"=1.0) -> ("高字节 2"=w15042:dbl, "高字节1"=w15044:dbl)  [unwired: 5 out]
                n5720 = call "输入分辨率计算-EV05.vi"("1字节?"=TRUE, "数值 2"=w15057, "数值"=w15058, "偏移量"=-40.0, "分辨率"=1.0) -> ("高字节 2"=w15052:dbl, "高字节1"=w15051:dbl)  [unwired: 5 out]
                n5721 = Build Array(w15051, w15052, w15045, w15043, w15044, w15042, w15041) -> (w15049:dbl[])
              }
              frame 5 {
                n5722 = Build Array(w15069) -> (w15066:dbl[])
              }
            }
          }
        }
        frame "通道电压节数" {
          n5723 = for {
            N: 1 -> [_]
            tunnel: [w15081] -> w15075 mode=indexing
            tunnel: [w15080] -> w15074 mode=indexing
            tunnel: [w15079] -> w15073 mode=indexing
            tunnel: w15072 -> [w15078]
            i -> [w15082]
            n5724 = case shown="0, 默认" w15082 {
              tunnel: w15078 -> [w15087]
              tunnel: [w15083] -> w15081
              tunnel: [w15085] -> w15080
              tunnel: [2 ("命令序号")] -> w15079
              frame 0, Default {
                w15085 = 20.0 ("y")
                n5725 = Unbundle By Name(w15087) -> ("项目信息 2"=w15088:refnum<vi>)
                n5726 = property class="Tbl (严格)"(reference=w15088) -> ("Value"=w15086:string[][])  [unwired: 1 in, 2 out]
                n5727 = Index Array(array=w15086, index (col)=1 ("禁用的索引 (列)")) -> (element=w15090:string[])  [unwired: 1 in]
                n5728 = Array Subset(array=w15090, index=22 ("索引"), length=w15085) -> (w15091:string[])
                n5729 = Fract/Exp String To Number(string=w15091) -> (number=w15084:dbl[])  [unwired: 4 out]
                n5730 = for {
                  tunnel: w15084 -> [w15095] mode=indexing
                  tunnel: [w15094] -> w15083 mode=indexing
                  w15096 = 12.0 ("y")
                  n5731 = Greater?(x=w15095, y=w15096) -> (0:w15097:bool)
                  n5732 = Select(t=w15096, s=w15097, f=w15095) -> (s? t:f=w15094:dbl)
                }
              }
            }
          }
        }
        frame "保险位置" {
          n5733 = for {
            N: 1 -> [_]
            tunnel: [w15109] -> w15103 mode=indexing
            tunnel: [w15108] -> w15102 mode=indexing
            tunnel: [w15107] -> w15101 mode=indexing
            tunnel: w15100 -> [w15106]
            i -> [w15110]
            n5734 = case shown="0, 默认" w15110 {
              tunnel: w15106 -> [w15117]
              tunnel: [w15111] -> w15109
              tunnel: [10.0 ("y")] -> w15108
              tunnel: [3 ("命令序号")] -> w15107
              frame 0, Default {
                n5735 = Unbundle By Name(w15117) -> ("项目信息 2"=w15118:refnum<vi>)
